vi "Read Camera Ini.vi"(11 "error in (no error)":errorcluster) -> (3 "CameraName":string, 4 "ROI":T4={"Global Rectangle"=[0, 0, 640, 480], "Contours"=[{"Contour Type"=0, "ROI Type"=3, "Points"=[4, 4, 636, 476]}]}, 6 "Image folder":path, 8 "File Type":T1, 10 "Image Save Rate (s)":dbl=10.0 format="%#_5f", 12 "Interface inputs":T3={"Elevation of top of Field of View (cm)"=10.0, "Field of View Height (cm)"=-0.1, "Smooth Length (cm)"=5.0, "Min derivative magnitude"=5.0, "Color Plane"=enum."Green"} {"Smooth Length (cm)" min=0.01 max=1000.0 step=0.1; "Field of View Height (cm)" min=0.1 max=1000.0 step=0.1}, 13 "Rotate":T2, 14 "Record images":bool, 15 "error out":errorcluster)   [LabVIEW 2019, in "Camera SubVIs.lvlib"]
uses:
  Camera SubVIs.lvlib
  <vilib>/Utility/config.llb/NI_LVConfig.lvlib
  <vilib>/Utility/config.llb/Read Key (String).vi
  <vilib>/Utility/config.llb/Read Key (Path).vi
  <vilib>/Utility/config.llb/Read Key (Double).vi
  <vilib>/Utility/config.llb/Read Key (Boolean).vi
  Calibration and Function folders.ctl
  <vilib>/Utility/config.llb/Read Key (I32).vi
  Image File Type.ctl
  Rotate.ctl
  Interface Inputs.ctl
panel:
  in  "Default Interface inputs":T3={"Elevation of top of Field of View (cm)"=10.0, "Field of View Height (cm)"=10.0, "Smooth Length (cm)"=0.1, "Min derivative magnitude"=1.0, "Color Plane"=enum."Combined"} {"Smooth Length (cm)" min=0.01 max=1000.0 step=0.1; "Field of View Height (cm)" min=0.1 max=1000.0 step=0.1}
  in  "Default ROI":T4={"Global Rectangle"=[0, 0, 640, 480], "Contours"=[{"Contour Type"=0, "ROI Type"=3, "Points"=[4, 4, 636, 476]}]}
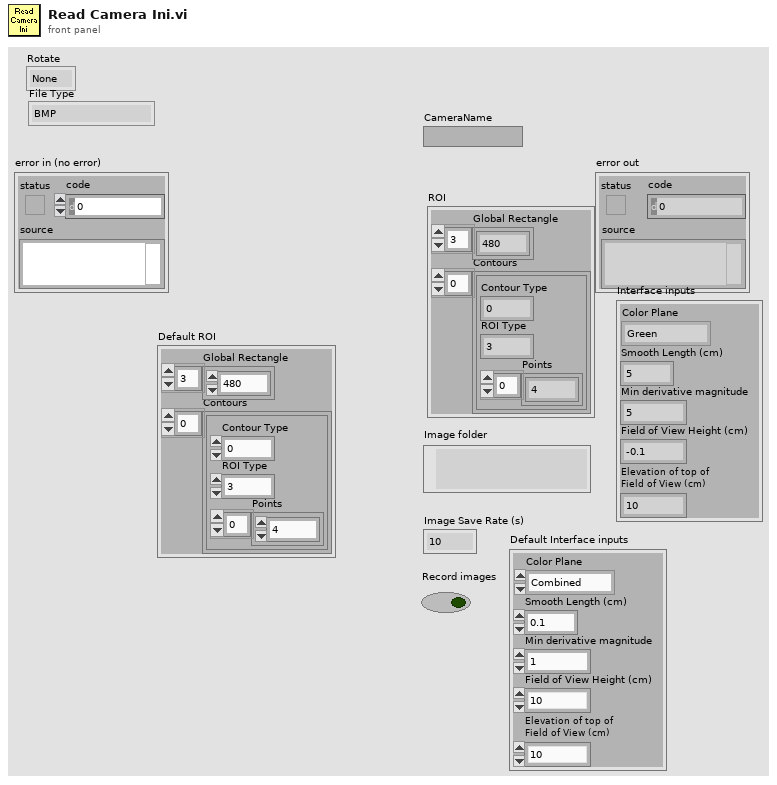
[diagram p1: front panel]
types:
  T1 = typedef "Camera SubVIs.lvlib/Image File Type.ctl" = enum16{"BMP", "JPEG", "JPEG 2000", "PNG", "PNG with Vision Info", "TIFF"}
  T2 = typedef "Camera SubVIs.lvlib/Rotate.ctl" = enum16{"None", "CW", "CCW"}
  T3 = typedef "Camera SubVIs.lvlib/Interface Inputs.ctl" = cluster{"Elevation of top of Field of View (cm)":dbl, "Field of View Height (cm)":dbl, "Smooth Length (cm)":dbl, "Min derivative magnitude":dbl, "Color Plane":enum16{"Red", "Green", "Blue", "Combined"}}
  T4 = cluster{"Global Rectangle":i32[], "Contours":cluster{"Contour Type":u32, "ROI Type":u32, "Points":i32[]}[]}
  T5 = typedef "Calibration and Function folders.ctl" = enum16{"Sensors", "Functions", "Config File", "PublicAppFolder", "New ini File", "Set Config File", "Delete ini File"}
  T6 = typedef "NI_LVConfig.lvlib/Config Data RefNum.ctl" = refnum<k1>
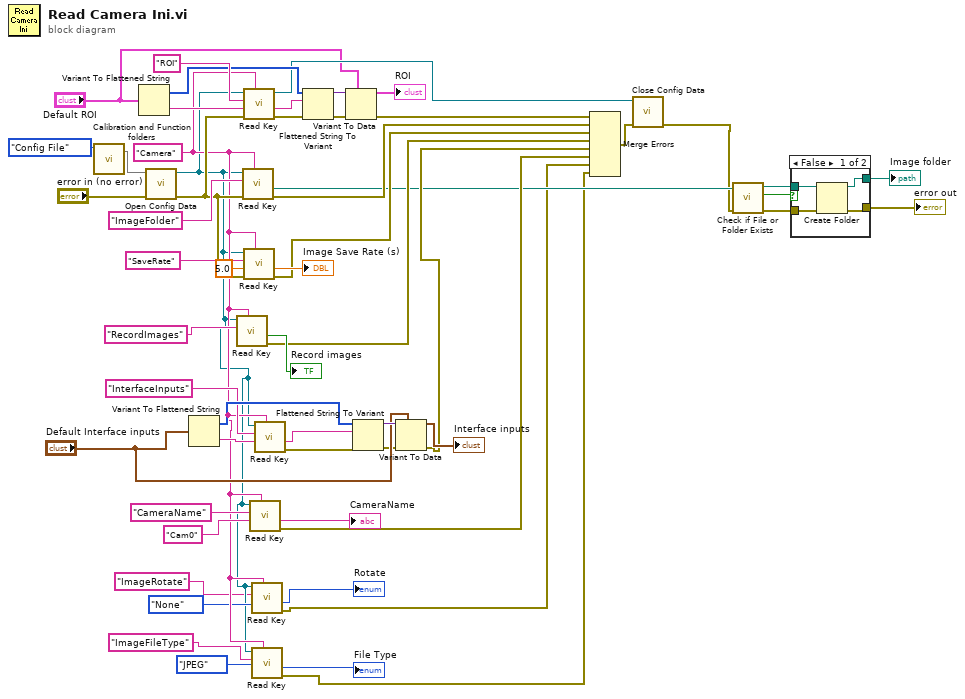
[diagram p0: block diagram]
diagram:
  w7 = "Camera" ("section")
  n1 = call "Calibration and Function folders.vi"(11:Calibration_and_Function_folders."Config File" ("Folder")) -> (7:w11)  [unwired: 8 in, 2 out]
  n2 = Variant To Flattened String(Variant="Default ROI") -> (data string=w55:string, 1:w54:i16[])
  n3 = call <vilib>:"Open Config Data.vi"("error in (no error)"="error in (no error)", "configuration file path"=w11) -> ("error out"=w43:errorcluster, "refnum"=w3:T6)  [unwired: 7 in, 1 out]
  n4 = Variant To Flattened String(Variant="Default Interface inputs") -> (data string=w33:string, 1:w34:i16[])
  n5 = call-poly <vilib>:"Read Key.vi"("section"=w7, "key"="RecordImages", "refnum"=w3) -> ("error out"=w36:errorcluster, "value"=→"Record images":bool)  [unwired: 5 in, 2 out]
  n6 = call-poly <vilib>:"Read Key.vi"("section"=w7, "error in (no error)"=w43, "key"="ImageFolder", "refnum"=w3) -> ("error out"=w41:errorcluster, "value"=w17:path)  [unwired: 4 in, 2 out]
  n7 = call-poly <vilib>:"Read Key.vi"("section"=w7, "error in (no error)"=w43, "default value"=w55, "key"="ROI", "refnum"=w3) -> ("error out"=w50:errorcluster, "value"=w53:string, "refnum out"=w49:T6)  [unwired: 3 in, 1 out]
  n8 = call-poly <vilib>:"Read Key.vi"("section"=w7, "error in (no error)"=w43, "default value"=5.0, "key"="SaveRate", "refnum"=w3) -> ("error out"=w40:errorcluster, "value"=→"Image Save Rate (s)":dbl)  [unwired: 3 in, 2 out]
  n9 = call-poly <vilib>:"Read Key.vi"("section"=w7, "default value"="Cam0", "key"="CameraName", "refnum"=w3) -> ("error out"=w21:errorcluster, "value"=→"CameraName":string)  [unwired: 4 in, 2 out]
  n10 = call-poly <vilib>:"Read Key.vi"("section"=w7, "default value"=Rotate."None" ("Rotate"), "key"="ImageRotate", "refnum"=w3) -> ("error out"=w5:errorcluster, "value"=→"Rotate":i32)  [unwired: 4 in, 2 out]
  n11 = call-poly <vilib>:"Read Key.vi"("section"=w7, "default value"=Image_File_Type."JPEG" ("File Type"), "key"="ImageFileType", "refnum"=w3) -> ("error out"=w4:errorcluster, "value"=→"File Type":i32)  [unwired: 4 in, 2 out]
  n12 = call-poly <vilib>:"Read Key.vi"("section"=w7, "default value"=w33, "key"="InterfaceInputs", "refnum"=w3) -> ("error out"=w27:errorcluster, "value"=w31:string)  [unwired: 4 in, 2 out]
  n13 = Flattened String To Variant(4:w50, 6:w53, 7:w54) -> (0:w51:errorcluster, 3:w52:variant)
  n14 = Variant To Data(error in=w51, type="Default ROI", Variant=w52) -> (data=→"ROI":T4, error out=w42:errorcluster)
  n15 = Flattened String To Variant(4:w27, 6:w31, 7:w34) -> (0:w26:errorcluster, 3:w30:variant)
  n16 = Variant To Data(error in=w26, type="Default Interface inputs", Variant=w30) -> (data=→"Interface inputs":T3, error out=w25:errorcluster)
  n17 = Merge Errors(w42, w41, w40, w36, w25, w21, w5, w4) -> (w39:errorcluster)
  n18 = call <vilib>:"Close Config Data.vi"("error in (no error)"=w39, "refnum"=w49) -> ("error out"=w16:errorcluster)  [unwired: 8 in, 1 out]
  n19 = call <vilib>:"Check if File or Folder Exists.vi"("error in (no error)"=w16, "path"=w17) -> ("error out"=w20:errorcluster, "file or folder exists?"=w18:bool, "dup path"=w19:path)  [unwired: 7 in]
  n20 = case shown="False" w18 {
    tunnel: w20 -> [w60 w62]
    tunnel: w19 -> [w59 w61]
    tunnel: [w58 w62] -> w15
    tunnel: [w57 w61] -> w14
    frame False {
      n21 = Create Folder(path (use dialog)=w59, error in=w60) -> (created path=w57:path, error out=w58:errorcluster)  [unwired: 1 in, 1 out]
    }
    frame True {
    }
  }
  "Image folder" <- w14
  "error out" <- w15
